vi "set_alarm.vi"(3 "audio":bool=TRUE, 4 "audio_alarm_interval":dbl=30.0, 5 "color":bool=TRUE, 6 "value_ref":refnum<vi>, 8 "time_last_audio_alarm_in":timestamp, 10 "warning":bool, 11 "error":bool) -> (0 "time_last_audio_alarm_out":timestamp)   [LabVIEW 2019]
panel:
  # "\"time_..._in\" and \"time_..._out\" must be connected\n via Feedback Node or Shift Register in a loop that calls this sub VI."
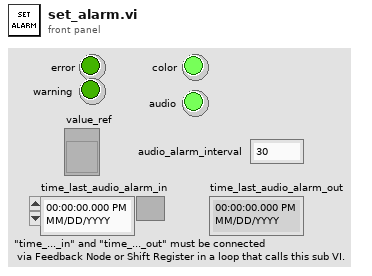
[diagram p1: front panel]
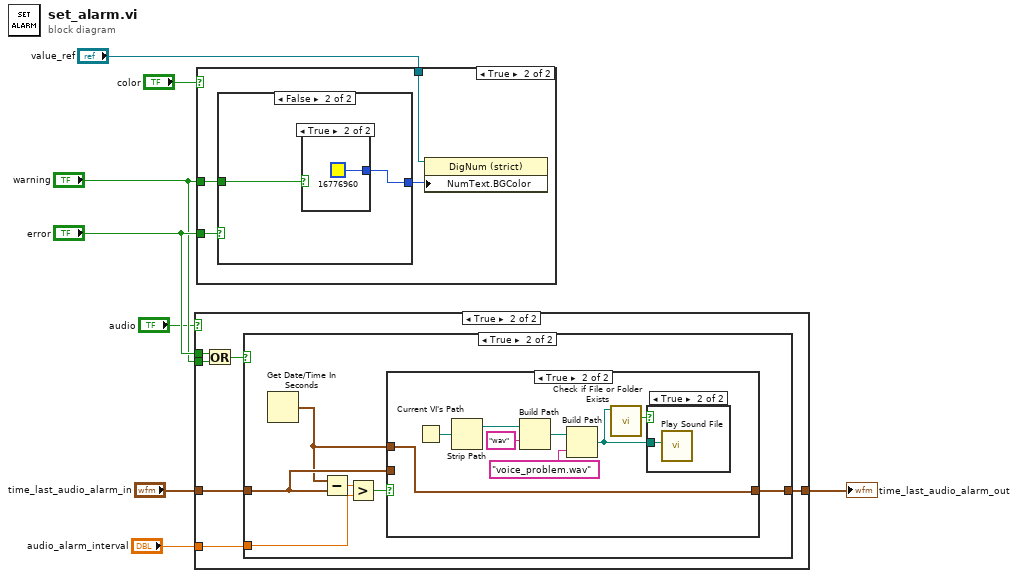
[diagram p0: block diagram]
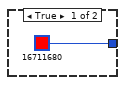
[diagram p7: hidden frame]
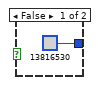
[diagram p8: hidden frame]
diagram:
  n1 = case shown="True" "audio" {
    tunnel: "error" -> [_ w15]
    tunnel: "warning" -> [_ w14]
    tunnel: [w9 w12] -> w3
    tunnel: "time_last_audio_alarm_in" -> [w9 w11]
    tunnel: "audio_alarm_interval" -> [_ w10]
    frame False {
    }
    frame True {
      n2 = Or(x=w15, y=w14) -> (x .or. y?=w13:bool)
      n3 = case shown="True" w13 {
        tunnel: [w16 w19] -> w12
        tunnel: w11 -> [w16 w18]
        tunnel: w10 -> [_ w21]
        frame False {
          # "Do nothing when warn = error = false."
        }
        frame True {
          n4 = Get Date/Time In Seconds() -> (seconds since 1Jan1904=w17:timestamp)
          n5 = Subtract(x=w17, y=w18) -> (x-y=w22:dbl)
          n6 = Greater?(x=w22, y=w21) -> (0:w20:bool)
          n7 = case shown="True" w20 {
            tunnel: [w23 w24] -> w19
            tunnel: w18 -> [w23 _]
            tunnel: w17 -> [_ w24]
            frame False {
            }
            frame True {
              n8 = Current VI's Path() -> (path=w31:path)
              n9 = Strip Path(path=w31) -> (stripped path=w30:path)  [unwired: 1 out]
              n10 = Build Path(base path=w30, name or relative path="wav") -> (appended path=w28:path)
              n11 = Build Path(base path=w28, name or relative path="voice_problem.wav") -> (appended path=w26:path)
              n12 = call <vilib>:"Check if File or Folder Exists.vi"("path"=w26) -> ("file or folder exists?"=w27:bool)  [unwired: 8 in, 2 out]
              n13 = case shown="True" w27 {
                tunnel: w26 -> [_ w32]
                frame False {
                }
                frame True {
                  n14 = call <vilib>:"Play Sound File.vi"("path"=w32) -> ()  [unwired: 9 in, 2 out]
                }
              }
            }
          }
        }
      }
    }
  }
  "time_last_audio_alarm_out" <- w3
  n15 = case shown="True" "color" {
    tunnel: "error" -> [_ w36]
    tunnel: "value_ref" -> [_ w35]
    tunnel: "warning" -> [_ w33]
    frame False {
    }
    frame True {
      n16 = case shown="False" w36 {
        tunnel: [u32 16711680 ("Numeric Text.Text Colors:BG Color") w39] -> w34
        tunnel: w33 -> [_ w38]
        frame True {
        }
        frame False {
          n17 = case shown="True" w38 {
            tunnel: [u32 13816530 ("Numeric Text.Text Colors:BG Color") u32 16776960 ("Numeric Text.Text Colors:BG Color")] -> w39
            frame False {
            }
            frame True {
            }
          }
        }
      }
      n18 = property on="Property Node" class="DigNum (strict)"(reference=w35, "NumText.BGColor"=w34) -> ()  [unwired: 1 in, 2 out]
    }
  }
